vi "UTILITY Log String to Spreadsheet.vi"(6 "String":string, 8 "error in (no error)":errorcluster, 9 "FileName":path) -> (0 "error out":errorcluster)   [LabVIEW 2016]
uses:
  <vilib>/Utility/file.llb/Write To Spreadsheet File (string).vi
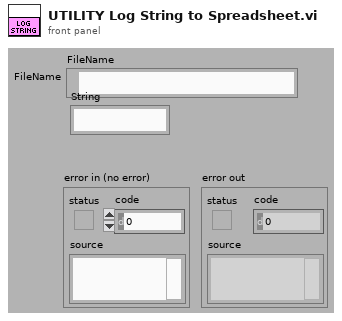
[diagram p1: front panel]
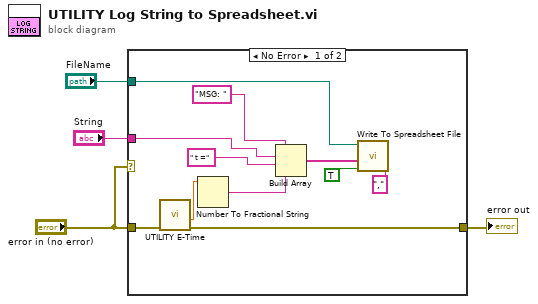
[diagram p0: block diagram]
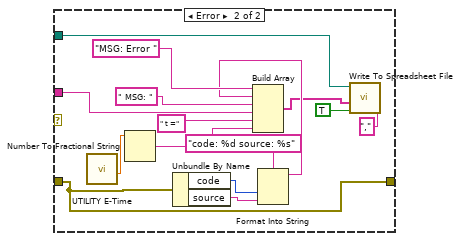
[diagram p2: hidden frame]
diagram:
  n1 = case shown="No Error" "error in (no error)" {
    tunnel: "error in (no error)" -> [w12 w24]
    tunnel: [w11 w24] -> w4
    tunnel: "FileName" -> [w7 w25]
    tunnel: "String" -> [w6 w17]
    frame No Error {
      n2 = call "UTILITY E-Time.vi"("error in (no error)"=w12) -> ("error out"=w11:errorcluster, "Elapsed Time (sec)"=w13:dbl)  [unwired: 8 in, 1 out]
      n3 = Number To Fractional String(number=w13) -> (F-format string=w8:string)  [unwired: 3 in]
      n4 = Build Array("MSG: " ("string"), w6, " t =" ("string"), w8) -> (w5:string[])
      n5 = call-poly <vilib>:"Write To Spreadsheet File.vi"("delimiter (\\t)"="," ("delimiter (\\t)"), "append to file? (new file:F)"=TRUE, "1D data"=w5, "file path (dialog if empty)"=w7) -> ()  [unwired: 4 in, 1 out]
    }
    frame Error {
      n6 = call "UTILITY E-Time.vi"() -> ("Elapsed Time (sec)"=w28:dbl)  [unwired: 9 in, 2 out]
      n7 = Number To Fractional String(number=w28) -> (F-format string=w26:string)  [unwired: 3 in]
      n8 = Unbundle By Name(w24) -> ("code"=w23:i32, "source"=w22:string)
      n9 = Format Into String(format string="code: %d source: %s", w23, w22) -> (resulting string=w19:string)  [unwired: 2 in, 1 out]
      n10 = Build Array("MSG: Error " ("string"), w19, " MSG: " ("string"), w17, " t =" ("string"), w26) -> (w16:string[])
      n11 = call-poly <vilib>:"Write To Spreadsheet File.vi"("delimiter (\\t)"="," ("delimiter (\\t)"), "append to file? (new file:F)"=TRUE, "1D data"=w16, "file path (dialog if empty)"=w25) -> ()  [unwired: 4 in, 1 out]
    }
  }
  "error out" <- w4
